vi "Get Path Tag.vi"(8 "error in (no error)":errorcluster, 10 "Tag Name":string, 11 "Log File Specification in":refnum<class "Log File Specification.lvclass">) -> (0 "error out":errorcluster, 1 "Tag Value":string, 3 "Log File Specification out":refnum<class "Log File Specification.lvclass">)   [LabVIEW 2015, in "Waveform Data Logger Shared.lvlib" / "Log File Specification.lvclass"]
uses:
  Log File Specification.lvclass
  Log File Specification.lvclass/Log File Specification.ctl
panel:
  out "Found":bool
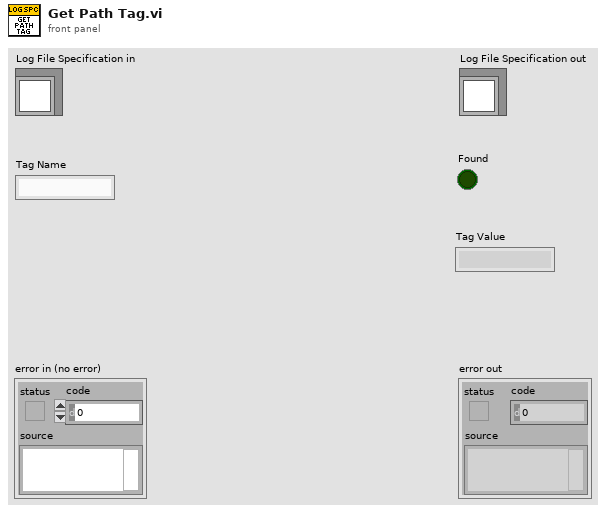
[diagram p1: front panel]
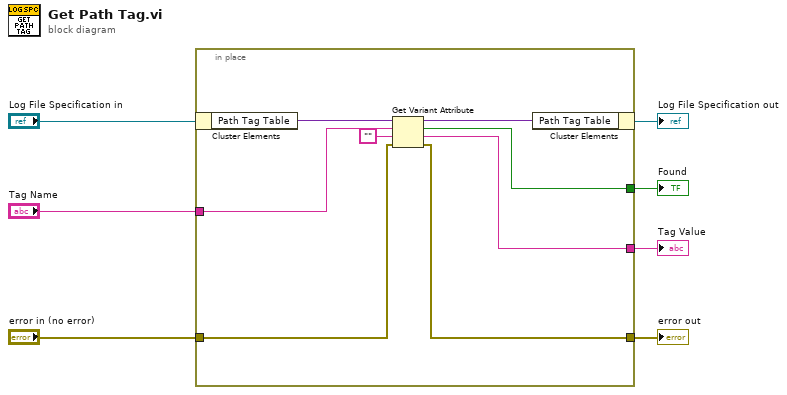
[diagram p0: block diagram]
diagram:
  n1 = in-place {
    in-place-border: "error in (no error)" -> [w13]
    in-place-border: [w12] -> w4
    in-place-border: "Tag Name" -> [w11]
    in-place-border: [w9] -> w2
    in-place-border: [w8] -> w1
    n2 = in-place-cluster #1("Log File Specification in") -> ("Path Tag Table"=w15:variant)
    n3 = Get Variant Attribute(Variant=w15, name=w11, default value (empty Variant)="", error in=w13) -> (duplicate Variant=w14:variant, found=w9:bool, value=w8:string, error out=w12:errorcluster)
    n4 = in-place-cluster #1("Path Tag Table"=w14) -> (→"Log File Specification out":refnum<class "Log File Specification.lvclass">)
  }
  "error out" <- w4
  "Tag Value" <- w1
  "Found" <- w2
